vi "XY Plot - Plot Area Width--Const.vi"() -> (3 "Plot Area:Size:Width":u32)   [LabVIEW 2017, in "DTacq Plot Display Library.lvlib"]
uses:
  DTacq Plot Display Library.lvlib
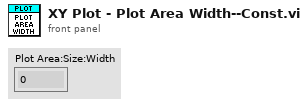
[diagram p1: front panel]
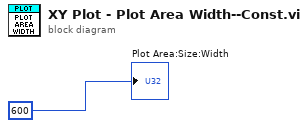
[diagram p0: block diagram]
diagram:
  "Plot Area:Size:Width" <- u32 600 ("Plot Area:Size:Width")
